vi "calc_dt_from_csv_col0_subvi.vi"(1 "array":dbl[](array[numeric])) -> (0 "dt":dbl)   [LabVIEW 2020]
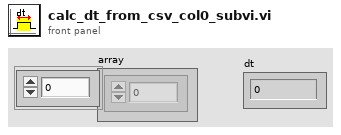
[diagram p1: front panel]
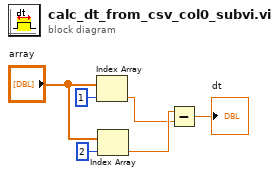
[diagram p0: block diagram]
diagram:
  n1 = Index Array(array="array", index=1) -> (element=w2:dbl)
  n2 = Index Array(array="array", index=2) -> (element=w3:dbl)
  n3 = Subtract(x=w3, y=w2) -> (x-y=→"dt":dbl)
